vi "Time_Select(SubVI).vi"(9 "error in (no error)":errorcluster, 10 "VISA resource name":refnum<visa-resource-name>, 11 "Array":bool[](array[boolean])) -> (0 "error out":errorcluster, 1 "ASCII string":string[](array[string]), 3 "Digital Outputs":bool[](array[boolean]), 5 "VISA resource name out":refnum<visa-resource-name>)   [LabVIEW 2022 SP3]
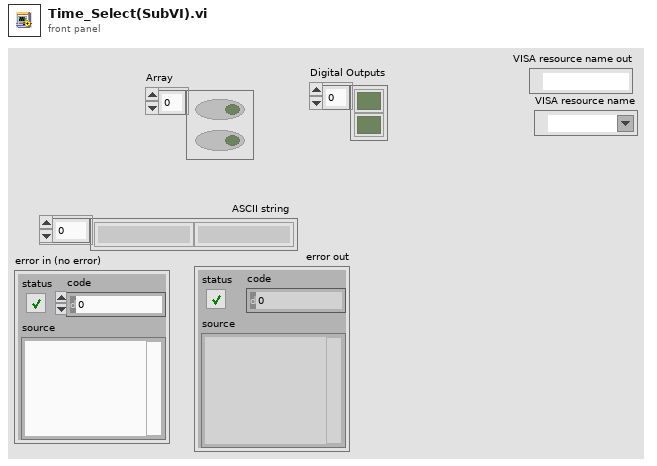
[diagram p1: front panel]
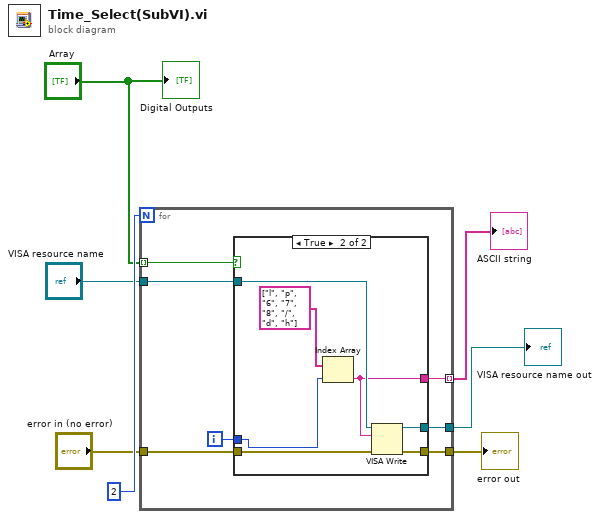
[diagram p0: block diagram]
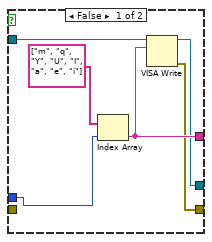
[diagram p2: hidden frame]
diagram:
  n1 = for {
    N: 2 -> [_]
    tunnel: "Array" -> [w14] mode=indexing
    tunnel: [w12] -> w7 mode=indexing
    tunnel: "VISA resource name" -> [w11]
    tunnel: [w10] -> w4
    tunnel: [w9] -> w3
    tunnel: "error in (no error)" -> [w8]
    i -> [w13]
    n2 = case shown="True" w14 {
      tunnel: w13 -> [w20 w26]
      tunnel: [w17 w24] -> w12
      tunnel: w11 -> [w18 w25]
      tunnel: [w16 w23] -> w10
      tunnel: [w15 w22] -> w9
      tunnel: w8 -> [_ w21]
      frame False {
        n3 = Index Array(array=string[] ["m", "q", "Y", "U", "I", "a", "e", "i"] ("ASCII LOW"), index=w20) -> (element=w17:string)
        n4 = VISA Write(VISA resource name=w18, write buffer=w17) -> (VISA resource name out=w16:refnum<visa-resource-name>, error out=w15:errorcluster)  [unwired: 1 in, 1 out]
      }
      frame True {
        n5 = Index Array(array=string[] ["l", "p", "6", "7", "8", "/", "d", "h"] ("ASCII HIGH"), index=w26) -> (element=w24:string)
        n6 = VISA Write(VISA resource name=w25, write buffer=w24, error in (no error)=w21) -> (VISA resource name out=w23:refnum<visa-resource-name>, error out=w22:errorcluster)  [unwired: 1 out]
      }
    }
  }
  "ASCII string" <- w7
  "VISA resource name out" <- w4
  "error out" <- w3
  "Digital Outputs" <- "Array"
